vi "General Setting Path to String.vi"(11 "General Setup (Path)":T1={"Export Path"=path "C:/Glass", "level"=0.8, "Time Gap"=20.0}) -> (3 "General Setup (String)":T2={"Export Path"="", "level"=0.8, "Time Gap"=20.0})   [LabVIEW 2015, in "ConfigHelper.lvlib"]
uses:
  ConfigHelper.lvlib
  Control_General Setup (String).ctl
  Control_General Setup (Path).ctl
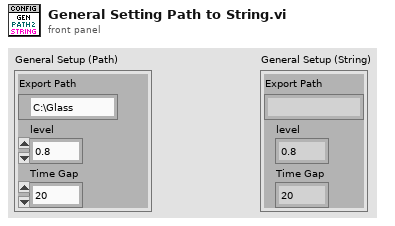
[diagram p1: front panel]
types:
  T1 = typedef "ConfigHelper.lvlib/Control_General Setup (Path).ctl" = cluster{"Export Path":path, "level":dbl, "Time Gap":dbl}
  T2 = typedef "ConfigHelper.lvlib/Control_General Setup (String).ctl" = cluster{"Export Path":string, "level":dbl, "Time Gap":dbl}
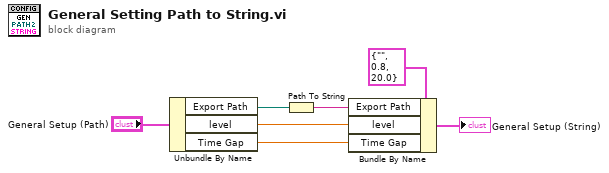
[diagram p0: block diagram]
diagram:
  n1 = Unbundle By Name("General Setup (Path)") -> ("Export Path"=w5:path, "level"=w2:dbl, "Time Gap"=w1:dbl)
  n2 = Path To String(path=w5) -> (string=w4:string)
  n3 = Bundle By Name(cluster=T2 {"Export Path"="", "level"=0.8, "Time Gap"=20.0} ("General Setup"), "Export Path"=w4, "level"=w2, "Time Gap"=w1) -> (→"General Setup (String)":T2)
